vi "v2.vi"() -> ()   [LabVIEW 2020]
uses:
  <vilib>/httpClient/PUTBuffer.vi
  <vilib>/httpClient/LabVIEWHTTPClient.lvlib
panel:
  out "error out":errorcluster
  in  "Simulate Pill Drop":bool
  out "Waveform Chart":dbl(graph)
  out "Temperature":dbl
  out "Pill Count":dbl
  out "DAQ Voltage":dbl
  out "Fan Trigger":bool
  out "Ready to Dispense":bool
  out "Temp Safe":bool
  out "Bottle Present":bool
  in  "Humidity":dbl(knob) scale=0.0..100.0
  in  "Temperature(C)":dbl(knob) scale=20.0..70.0 scale format="%#_2g"
  in  "Bottle Weight(g)":dbl(slide) scale=0.0..500.0
  in  "stop":bool
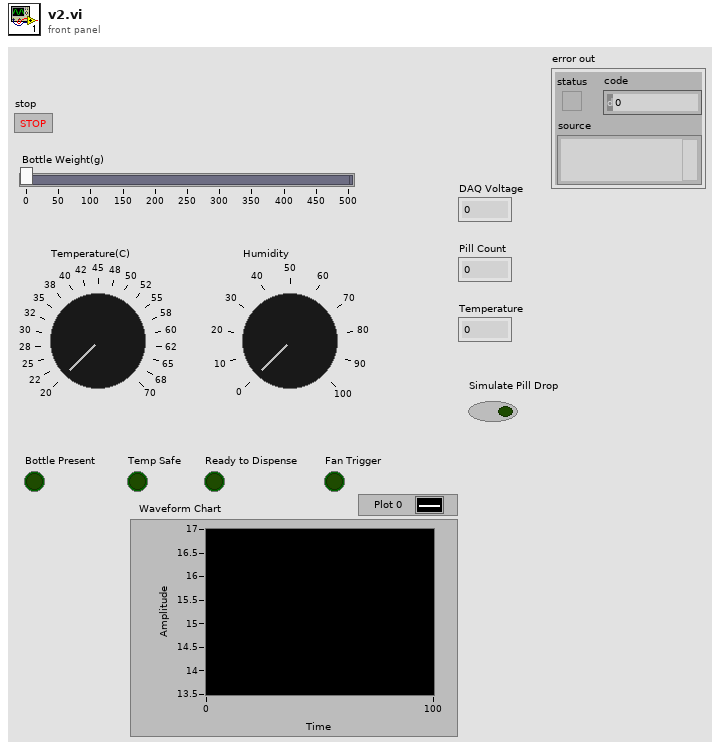
[diagram p1: front panel]
types:
  T1 = typedef "LabVIEWHTTPClient.lvlib/ClientHandle.ctl" = refnum<k1>
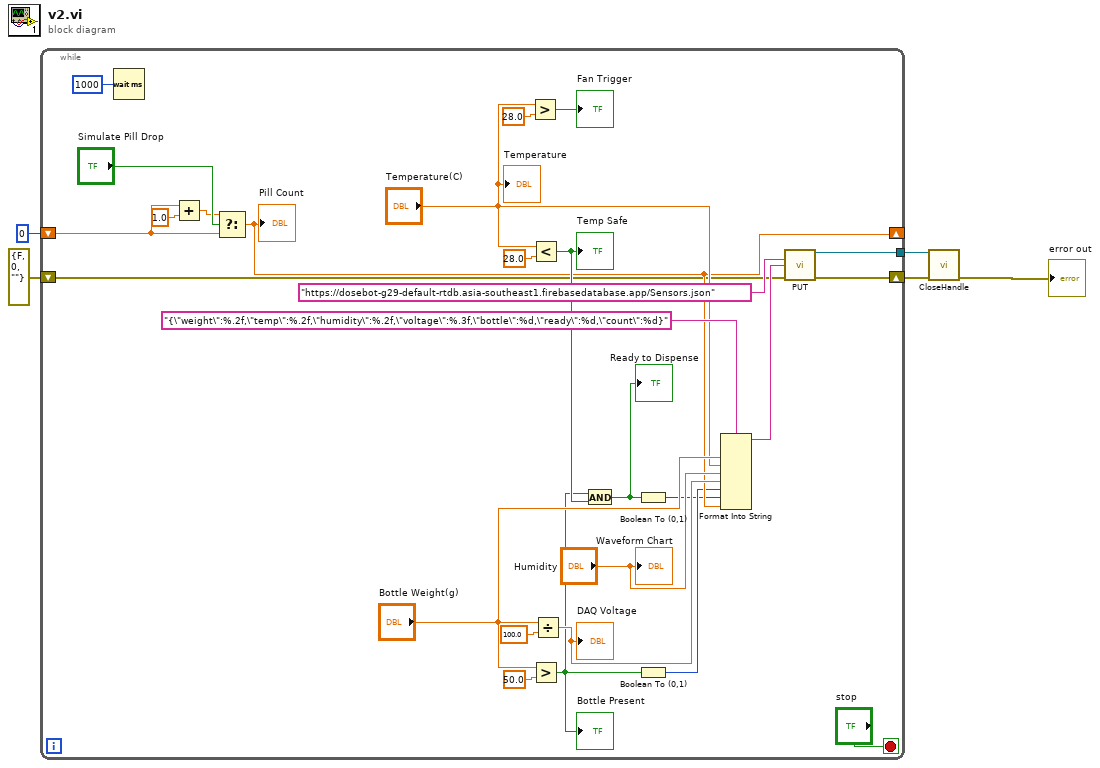
[diagram p0: block diagram]
diagram:
  n1 = while {
    shift-right: [w15] -> _
    shift-left: 0 -> [w21]
    shift-right: [w12] -> w4
    shift-left: errorcluster {"status"=FALSE, "code"=0, "source"=""} ("error out") -> [w10]
    tunnel: [w11] -> w2
    stop <- "stop" stop-if-true
    n2 = Wait (ms)(milliseconds to wait=u32 1000) -> ()  [unwired: 1 out]
    n3 = Add(x=w21, y=1.0) -> (x+y=w22:dbl)
    n4 = Select(t=w22, s="Simulate Pill Drop", f=w21) -> (s? t:f=w15:dbl)
    "Pill Count" <- w15
    n5 = Greater?(x="Temperature(C)", y=28.0) -> (0:→"Fan Trigger":bool)
    n6 = Less?(x="Temperature(C)", y=28.0) -> (x < y?=w26:bool)
    "Temp Safe" <- w26
    n7 = Greater?(x="Bottle Weight(g)", y=50.0) -> (0:w9:bool)
    "Bottle Present" <- w9
    n8 = Divide(x="Bottle Weight(g)", y=100.0) -> (x/y=w16:dbl)
    "DAQ Voltage" <- w16
    n9 = And(x=w9, y=w26) -> (x .and. y?=w7:bool)
    "Ready to Dispense" <- w7
    n10 = Boolean To (0,1)(Boolean=w7) -> (0, 1=w6:i16)
    n11 = Boolean To (0,1)(Boolean=w9) -> (0, 1=w8:i16)
    n12 = Format Into String(format string="{\"weight\":%.2f,\"temp\":%.2f,\"humidity\":%.2f,\"voltage\":%.3f,\"bottle\":%d,\"ready\":%d,\"count\":%d}", "Bottle Weight(g)", "Temperature(C)", "Humidity", w16, w8, w6, w15) -> (resulting string=w13:string)  [unwired: 2 in, 1 out]
    n13 = call-poly <vilib>:"PUT.vi"("url"="https://dosebot-g29-default-rtdb.asia-southeast1.firebasedatabase.app/Sensors.json", "buffer"=w13, "error in (no error)"=w10) -> ("client handle out"=w11:T1, "error out"=w12:errorcluster)  [unwired: 9 in, 2 out]
    "Temperature" <- "Temperature(C)"
    "Waveform Chart" <- "Humidity"
  }
  n14 = call <vilib>:"CloseHandle.vi"("client handle"=w2, "error in (no error)"=w4) -> ("error out"=→"error out":errorcluster)  [unwired: 13 in]
